vi "Write DBL.vi"(8 "error in":errorcluster, 10 "Value":variant, 11 "TDMS Sink in":refnum<class "TDMS Sink.lvclass">) -> (0 "error out":errorcluster, 3 "TDMS Sink out":refnum<class "TDMS Sink.lvclass">)   [LabVIEW 2024, in "TDMS Sink.lvclass"]
uses:
  TDMS Sink.lvclass
  TDMS Sink.lvclass/TDMS Sink.ctl
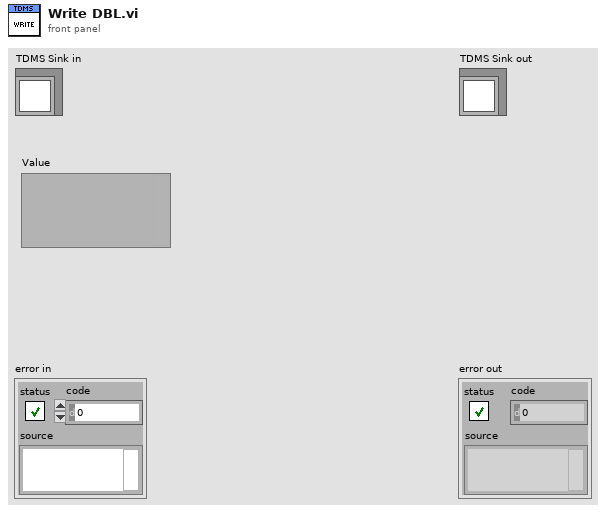
[diagram p1: front panel]
types:
  T1 = cluster{"Group":string, "Channels":string[], "Data":dbl[]}
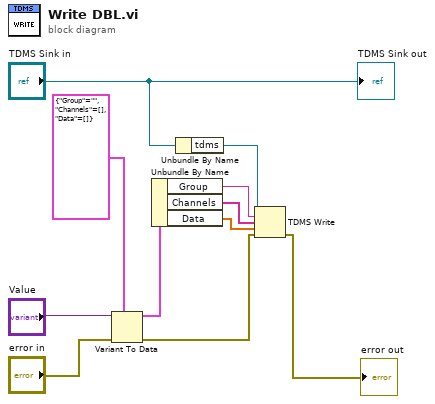
[diagram p0: block diagram]
diagram:
  n1 = Variant To Data(error in="error in", type=T1 {"Group"="", "Channels"=[], "Data"=[]}, Variant="Value") -> (data=w8:T1, error out=w5:errorcluster)
  n2 = Unbundle By Name(w8) -> ("Group"=w4:string, "Channels"=w3:string[], "Data"=w2:dbl[])
  n3 = Unbundle By Name("TDMS Sink in") -> ("tdms"=w6:refnum<k34>)
  n4 = TDMS Write(0:w6, 5:w4, 7:w3, 9:w2, 11:w5) -> (15:→"error out":errorcluster)  [unwired: 1 in, 3 out]
  "TDMS Sink out" <- "TDMS Sink in"
